vi "cycle ratio.vi"(1 "Stable Counts":dbl, 2 "rare Counts":dbl) -> (0 "Cycle ratio":dbl)   [LabVIEW 2016]
doc: "This calculates the value of the cycle ratio"
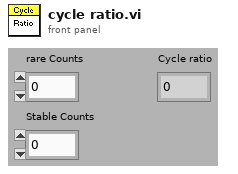
[diagram p1: front panel]
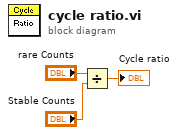
[diagram p0: block diagram]
diagram:
  n1 = Divide(x="rare Counts", y="Stable Counts") -> (x/y=→"Cycle ratio":dbl)
